vi "HEX string creator.vi"(1 "Destination address LSB":string="\u0001", 2 "Command":string="\u0000") -> (0 "String to send":string)   [LabVIEW 2013]
panel:
  out "Checksum":string
  in  "Options":string="\u0000"
  in  "Destination address MSB":string="P"
  in  "Frame ID":string="\u0001"
  in  "API identifier":string="\u0001"
  in  "Length LSB":string="\u0010"
  in  "Length MSB":string="\u0000"
  in  "Start delimeter":string="~"
  # "Example (send 100 to 5001)\n7E00 0901 0150 0100 3130 300D 0E"
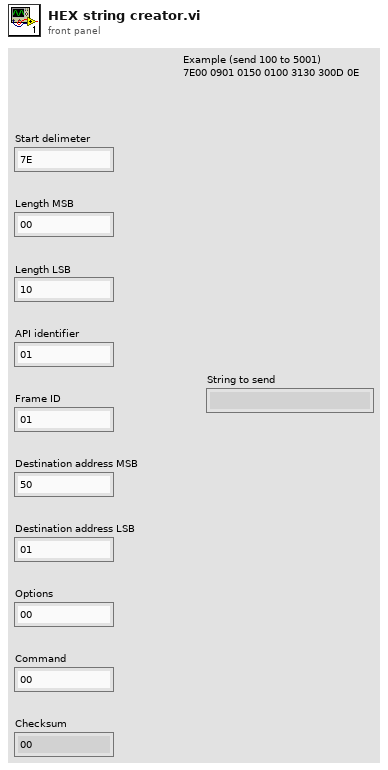
[diagram p1: front panel]
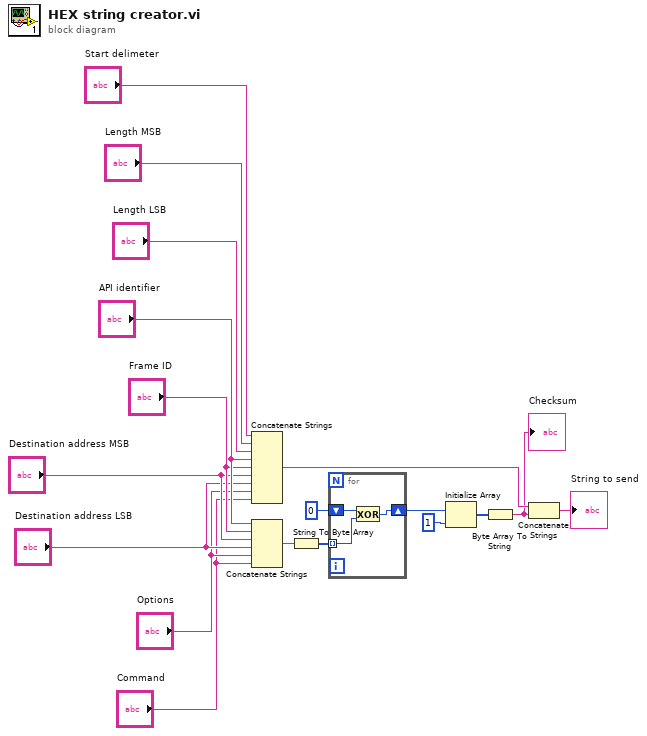
[diagram p0: block diagram]
diagram:
  n1 = Concatenate Strings("Start delimeter", "Length MSB", "Length LSB", "API identifier", "Frame ID", "Destination address MSB", "Destination address LSB", "Options", "Command") -> (w8:string)
  n2 = Concatenate Strings("API identifier", "Frame ID", "Destination address MSB", "Destination address LSB", "Options", "Command") -> (w7:string)
  n3 = String To Byte Array(string=w7) -> (unsigned byte array=w15:u8[])
  n4 = for {
    tunnel: w15 -> [w20] mode=indexing
    shift-right: [w21] -> w3
    shift-left: u8 0 -> [w19]
    n5 = Exclusive Or(1:w20, 2:w19) -> (0:w21:u8)
  }
  n6 = Initialize Array(w3, 1 ("dimension size")) -> (w2:u8[])
  n7 = Byte Array To String(unsigned byte array=w2) -> (string=w1:string)
  "Checksum" <- w1
  n8 = Concatenate Strings(w8, w1) -> (→"String to send":string)
